vi "Part 1.vi"(11 "Input":string) -> (3 "Output":i64)   [LabVIEW 2021]
uses:
  <userlib>/_OpenG.lib/string/string.llb/Convert EOLs (String)__ogtk.vi
panel:
  out "SNAFU Number":string
  # "2-20===01--222-0-0=2"
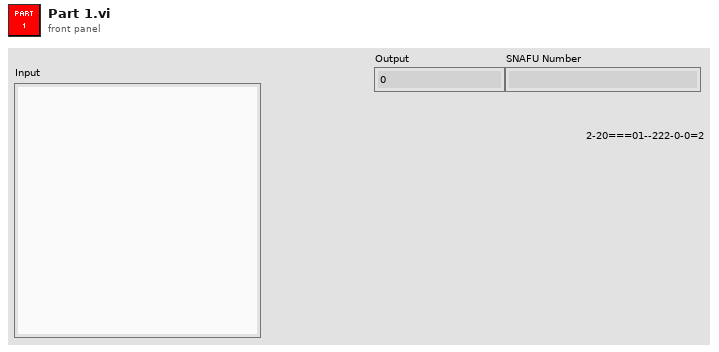
[diagram p1: front panel]
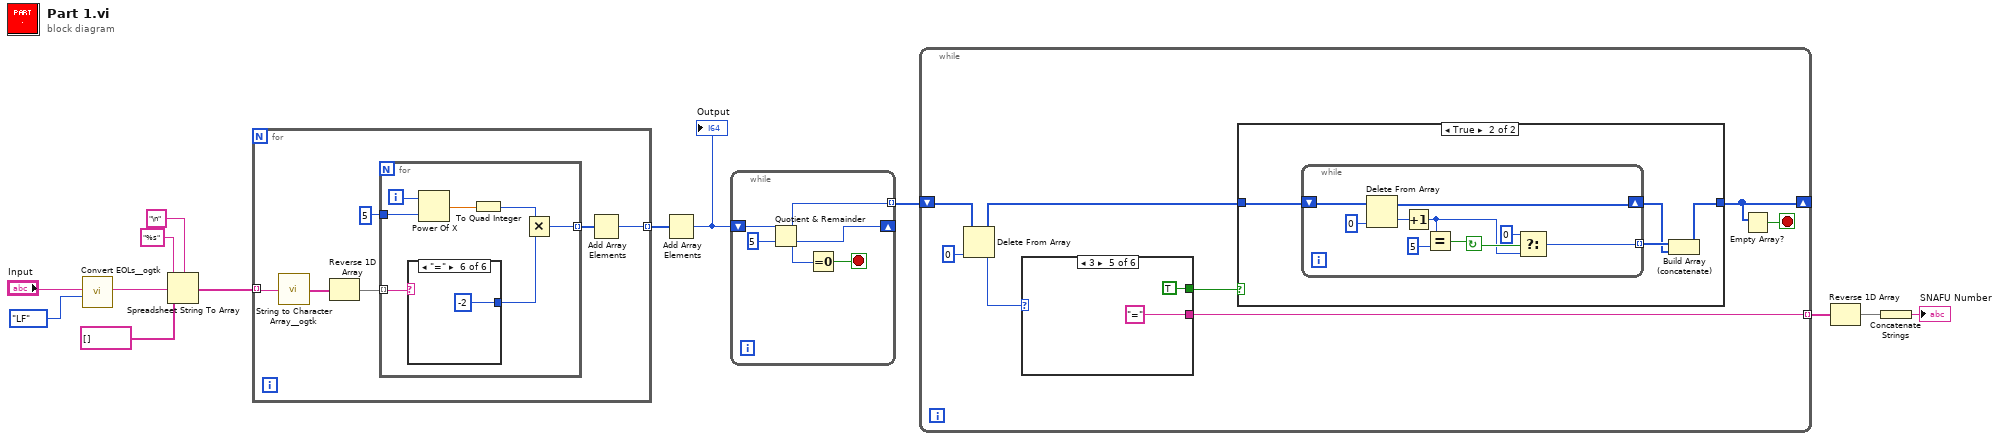
[diagram p0: block diagram]
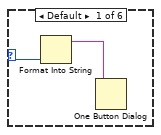
[diagram p3: hidden frame]
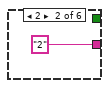
[diagram p4: hidden frame]
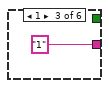
[diagram p5: hidden frame]
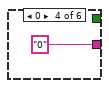
[diagram p6: hidden frame]
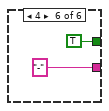
[diagram p7: hidden frame]
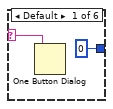
[diagram p8: hidden frame]
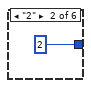
[diagram p9: hidden frame]
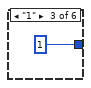
[diagram p10: hidden frame]
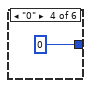
[diagram p11: hidden frame]
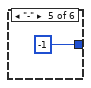
[diagram p12: hidden frame]
diagram:
  n1 = call-poly <userlib>:"Convert EOLs__ogtk.vi"("Convert to:"=enum16{"CR", "LF", "CRLF"}."LF", "String in"="Input") -> ("String out"=w9:string)  [unwired: 9 in]
  n2 = Spreadsheet String To Array(delimiter (Tab)="\n", format string="%s", spreadsheet string=w9, array type (2D Dbl)=string[] []) -> (array=w7:string[])
  n3 = for {
    tunnel: w7 -> [w19] mode=indexing
    tunnel: [w14] -> w6 mode=indexing
    n4 = call <userlib>:"String to Character Array__ogtk.vi"("Input String"=w19) -> ("Character Array"=w18:string[])
    n5 = Reverse 1D Array(array=w18) -> (reversed array=w17:string[])
    n6 = for {
      tunnel: w17 -> [w25] mode=indexing
      tunnel: 5 -> [w26]
      tunnel: [w22] -> w15 mode=indexing
      i -> [w21]
      n7 = case shown="\"=\"" w25 {
        selector: w25 -> [w28 _ _ _ _ _]
        tunnel: [0 2 1 0 -1 -2] -> w23
        frame Default {
          n8 = One Button Dialog(message=w28) -> ()  [unwired: 1 in, 1 out]
        }
        frame "2" {
        }
        frame "1" {
        }
        frame "0" {
        }
        frame "-" {
        }
        frame "=" {
        }
      }
      n9 = Power Of X(1:w26, 2:w21) -> (0:w24:dbl)
      n10 = To Quad Integer(1:w24) -> (0:w20:i64)
      n11 = Multiply(x=w20, y=w23) -> (x*y=w22:i64)
    }
    n12 = Add Array Elements(numeric array=w15) -> (sum=w14:i64)
  }
  n13 = Add Array Elements(numeric array=w6) -> (sum=w5:i64)
  "Output" <- w5
  n14 = while {
    shift-right: [w35] -> _
    shift-left: w5 -> [w38]
    tunnel: [w34] -> w4 mode=indexing
    stop <- w36 stop-if-true
    n15 = Quotient & Remainder(x=w38, y=i64 5) -> (x-y*floor(x/y)=w34:i64, floor(x/y)=w35:i64)
    n16 = Equal To 0?(x=w35) -> (x = 0?=w36:bool)
  }
  n17 = while {
    shift-right: [w40] -> _
    shift-left: w4 -> [w46]
    tunnel: [w43] -> w3 mode=indexing
    stop <- w39 stop-if-true
    n18 = Delete From Array(array=w46, index=0) -> (deleted portion=w44:i64, array with subset deleted=w41:i64[])  [unwired: 1 in]
    n19 = case shown="3" w44 {
      selector: w44 -> [w62 _ _ _ _ _]
      tunnel: [_ "2" "1" "0" "=" "-"] -> w43
      tunnel: [_ _ _ _ TRUE TRUE] -> w42
      frame Default {
        n20 = Format Into String(w62) -> (resulting string=w61:string)  [unwired: 3 in, 1 out]
        n21 = One Button Dialog(message=w61) -> ()  [unwired: 1 in, 1 out]
      }
      frame 2 {
      }
      frame 1 {
      }
      frame 0 {
      }
      frame 3 {
      }
      frame 4 {
      }
    }
    n22 = case shown="True" w42 {
      tunnel: w41 -> [w47 w51]
      tunnel: [w47 w48] -> w40
      frame False {
      }
      frame True {
        n23 = while {
          shift-right: [w57] -> w49
          shift-left: w51 -> [w60]
          tunnel: [w52] -> w50 mode=indexing
          stop <- w55 continue-if-true
          n24 = Delete From Array(array=w60, index=0) -> (deleted portion=w58:i64, array with subset deleted=w57:i64[])  [unwired: 1 in]
          n25 = Increment(x=w58) -> (x+1=w54:i64)
          n26 = Equal?(x=w54, y=i64 5) -> (x = y?=w55:bool)
          n27 = Select(t=i64 0, s=w55, f=w54) -> (s? t:f=w52:i64)
        }
        n28 = Build Array (concatenate)(w50, w49) -> (w48:i64[])
      }
    }
    n29 = Empty Array?(array=w40) -> (empty?=w39:bool)
  }
  n30 = Reverse 1D Array(array=w3) -> (reversed array=w2:string[])
  n31 = Concatenate Strings(w2) -> (→"SNAFU Number":string)
